vi "check_sweep.vi"() -> ()   [LabVIEW 2013]
uses:
  check_sweep_st_ma.ctl
  <vilib>/DAQmx/write.llb/DAQmx Write (Analog Wfm 1Chan NSamp).vi
  <vilib>/DAQmx/create/channels.llb/DAQmx Create Channel (AO-Voltage-Basic).vi
  <vilib>/DAQmx/configure/timing.llb/DAQmx Timing (Use Waveform).vi
  <vilib>/DAQmx/miscellaneous.llb/DAQmx Fill In Error Info.vi
panel:
  out "DAC_status":bool
  in  "RF address":string="19"
  in  "amplitude (mV)":i32=5
  in  "modulation (kHz)":i32=50
  in  "center frequency (MHz)":dbl=32.7
  in  "stop_daq":bool
  in  "start_daq":bool
  in  "init_daq":bool
  in  "rf_off":bool
  in  "rf_on":bool
  in  "set_rf":bool
  in  "Exit":bool
  in  "T":dbl=0.5
  in  "N_steps_1":i32=500 min=0 step=1
  in  "DAC channel":tag="Dev1/ao0"
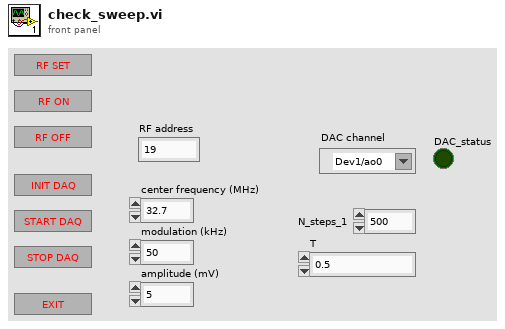
[diagram p1: front panel]
types:
  T1 = typedef "check_sweep_st_ma.ctl" = enum16{"exit", "idle", "init_daq", "start_daq", "stop_daq", "rf_off", "rf_on", "set_rf"}
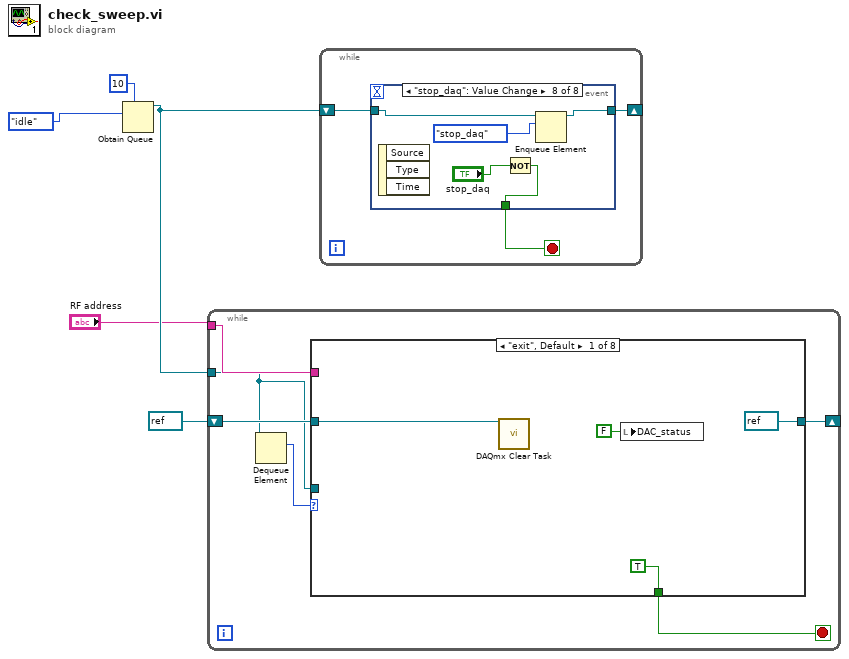
[diagram p0: block diagram]
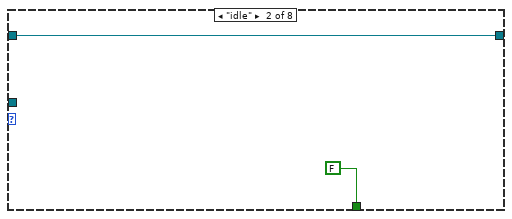
[diagram p2: hidden frame]
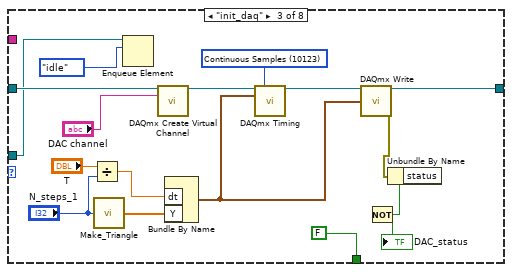
[diagram p3: hidden frame]
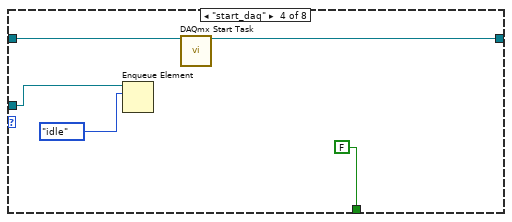
[diagram p4: hidden frame]
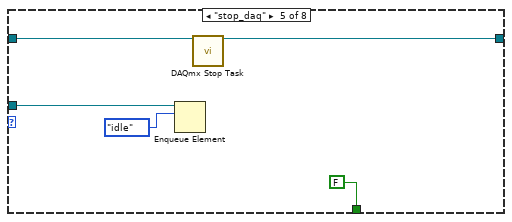
[diagram p5: hidden frame]
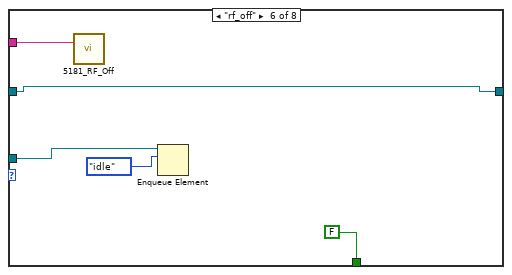
[diagram p6: hidden frame]
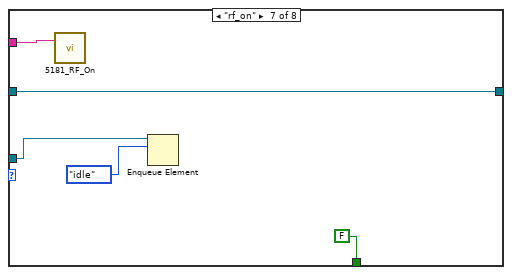
[diagram p7: hidden frame]
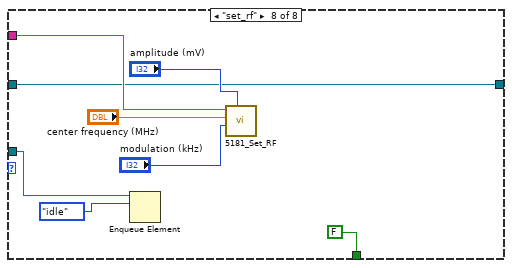
[diagram p8: hidden frame]
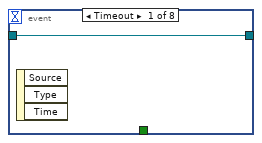
[diagram p9: hidden frame]
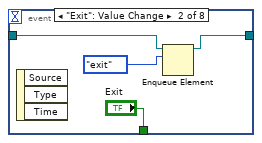
[diagram p10: hidden frame]
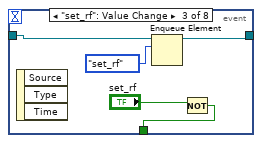
[diagram p11: hidden frame]
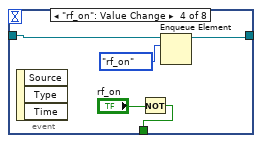
[diagram p12: hidden frame]
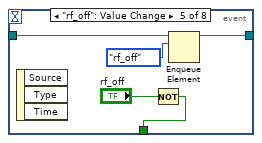
[diagram p13: hidden frame]
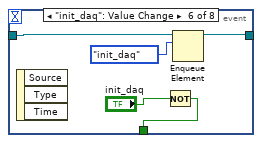
[diagram p14: hidden frame]
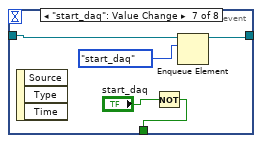
[diagram p15: hidden frame]
diagram:
  n1 = Obtain Queue(max queue size (-1, unlimited)=10, element data type=check_sweep_st_ma."idle") -> (queue out=w3:refnum<queue>)  [unwired: 3 in, 2 out]
  n2 = while {
    tunnel: w3 -> [w7]
    tunnel: "RF address" -> [w10]
    shift-right: [w9] -> _
    shift-left: refnum<k21> refnum ("task out") -> [w8]
    stop <- w6 stop-if-true
    n3 = Dequeue Element(queue=w7) -> (element=w11:T1)  [unwired: 2 in, 3 out]
    n4 = case shown="\"exit\", Default" w11 {
      tunnel: w10 -> [_ _ _ _ _ w49 w54 w60]
      tunnel: [refnum<k21> refnum ("task out") w17 w26 w38 w43 w48 w53 w58] -> w9
      tunnel: w8 -> [w15 w17 w24 w39 w44 w48 w53 w58]
      tunnel: w7 -> [_ _ w23 w37 w41 w46 w51 w57]
      tunnel: [TRUE FALSE FALSE FALSE FALSE FALSE FALSE FALSE] -> w6
      frame "exit", Default {
        n5 = call <vilib>:"DAQmx Clear Task.vi"("task in"=w15) -> ()  [unwired: 14 in, 1 out]
        n6 = local write "DAC_status"(FALSE ("DAC_status")) -> ()
      }
      frame "idle" {
      }
      frame "init_daq" {
        w30 = 10123 items=["Finite Samples"=10178, "Continuous Samples"=10123, "Hardware Timed Single Point"=12522] ("sample mode")
        n7 = Divide(x="T", y="N_steps_1") -> (x/y=w34:dbl)
        n8 = call "Make_Triangle.vi"("N_steps_1"="N_steps_1") -> ("TriangleWaveform"=w32:dbl[])
        n9 = Enqueue Element(queue=w23, element=check_sweep_st_ma."idle") -> ()  [unwired: 2 in, 3 out]
        n10 = call-poly <vilib>:"DAQmx Create Virtual Channel.vi"("task in"=w24, "physical channels"="DAC channel") -> ("task out"=w27:refnum<k21>)  [unwired: 12 in, 1 out]
        n11 = Bundle By Name("dt"=w34, "Y"=w32) -> (w28:waveform(dbl))  [unwired: 1 in]
        n12 = call-poly <vilib>:"DAQmx Timing.vi"("task/channels in"=w27, "sample mode"=w30, "waveform"=w28) -> ("task out"=w29:refnum<k21>)  [unwired: 11 in, 1 out]
        n13 = call-poly <vilib>:"DAQmx Write.vi"("task/channels in"=w29, "data"=w28) -> ("task out"=w26:refnum<k21>, "error out"=w18:errorcluster)  [unwired: 11 in, 1 out]
        n14 = Unbundle By Name(w18) -> ("status"=w20:bool)
        n15 = Not(x=w20) -> (.not. x?=→"DAC_status":bool)
      }
      frame "start_daq" {
        n16 = Enqueue Element(queue=w37, element=check_sweep_st_ma."idle") -> ()  [unwired: 2 in, 3 out]
        n17 = call <vilib>:"DAQmx Start Task.vi"("task/channels in"=w39) -> ("task out"=w38:refnum<k21>)  [unwired: 13 in, 1 out]
      }
      frame "stop_daq" {
        n18 = Enqueue Element(queue=w41, element=check_sweep_st_ma."idle") -> ()  [unwired: 2 in, 3 out]
        n19 = call <vilib>:"DAQmx Stop Task.vi"("task/channels in"=w44) -> ("task out"=w43:refnum<k21>)  [unwired: 13 in, 1 out]
      }
      frame "rf_off" {
        n20 = call "5181_RF_Off.vi"("address"=w49) -> ()  [unwired: 1 in, 2 out]
        n21 = Enqueue Element(queue=w46, element=check_sweep_st_ma."idle") -> ()  [unwired: 2 in, 3 out]
      }
      frame "rf_on" {
        n22 = call "5181_RF_On.vi"("address"=w54) -> ()  [unwired: 1 in, 2 out]
        n23 = Enqueue Element(queue=w51, element=check_sweep_st_ma."idle") -> ()  [unwired: 2 in, 3 out]
      }
      frame "set_rf" {
        n24 = Enqueue Element(queue=w57, element=check_sweep_st_ma."idle") -> ()  [unwired: 2 in, 3 out]
        n25 = call "5181_Set_RF.vi"("address"=w60, "center frequency (MHz)"="center frequency (MHz)", "modulation (kHz)"="modulation (kHz)", "amplitude (mV)"="amplitude (mV)") -> ()  [unwired: 1 in, 2 out]
      }
    }
  }
  n26 = while {
    shift-right: [w63] -> _
    shift-left: w3 -> [w64]
    stop <- w65 stop-if-true
    n27 = event shown="[7] \"stop_daq\": Value Change" {
      selector: _ -> [_ _ _ _ _ _ _ _]
      dyn-events: _ -> [_ _ _ _ _ _ _ _]
      timeout: _ -> [_ _ _ _ _ _ _ _]
      tunnel: [_ "Exit" w72 w77 w82 w87 w92 w98] -> w65
      tunnel: w64 -> [w66 w69 w75 w80 w85 w90 w95 w100]
      tunnel: [w66 w68 w74 w79 w84 w89 w94 w99] -> w63
      event Timeout {
        n28 = event-data() -> ()  [unwired: 1 in, 3 out]
      }
      event "Exit": Value Change {
        n29 = event-data() -> ()  [unwired: 1 in, 3 out]
        n30 = Enqueue Element(queue=w69, element=check_sweep_st_ma."exit") -> (queue out=w68:refnum<queue>)  [unwired: 2 in, 2 out]
      }
      event "set_rf": Value Change {
        n31 = event-data() -> ()  [unwired: 1 in, 3 out]
        n32 = Enqueue Element(queue=w75, element=check_sweep_st_ma."set_rf") -> (queue out=w74:refnum<queue>)  [unwired: 2 in, 2 out]
        n33 = Not(x="set_rf") -> (.not. x?=w72:bool)
      }
      event "rf_on": Value Change {
        n34 = event-data() -> ()  [unwired: 1 in, 3 out]
        n35 = Not(x="rf_on") -> (.not. x?=w77:bool)
        n36 = Enqueue Element(queue=w80, element=check_sweep_st_ma."rf_on") -> (queue out=w79:refnum<queue>)  [unwired: 2 in, 2 out]
      }
      event "rf_off": Value Change {
        n37 = event-data() -> ()  [unwired: 1 in, 3 out]
        n38 = Not(x="rf_off") -> (.not. x?=w82:bool)
        n39 = Enqueue Element(queue=w85, element=check_sweep_st_ma."rf_off") -> (queue out=w84:refnum<queue>)  [unwired: 2 in, 2 out]
      }
      event "init_daq": Value Change {
        n40 = event-data() -> ()  [unwired: 1 in, 3 out]
        n41 = Not(x="init_daq") -> (.not. x?=w87:bool)
        n42 = Enqueue Element(queue=w90, element=check_sweep_st_ma."init_daq") -> (queue out=w89:refnum<queue>)  [unwired: 2 in, 2 out]
      }
      event "start_daq": Value Change {
        n43 = event-data() -> ()  [unwired: 1 in, 3 out]
        n44 = Not(x="start_daq") -> (.not. x?=w92:bool)
        n45 = Enqueue Element(queue=w95, element=check_sweep_st_ma."start_daq") -> (queue out=w94:refnum<queue>)  [unwired: 2 in, 2 out]
      }
      event "stop_daq": Value Change {
        n46 = event-data() -> ()  [unwired: 1 in, 3 out]
        n47 = Not(x="stop_daq") -> (.not. x?=w98:bool)
        n48 = Enqueue Element(queue=w100, element=check_sweep_st_ma."stop_daq") -> (queue out=w99:refnum<queue>)  [unwired: 2 in, 2 out]
      }
    }
  }
